vi "CallEngine.vi"(8 "error in (no error)":errorcluster, 10 "RT_Game.lvlib:Engine.lvclass":refnum<class "Engine.lvclass">, 11 "SnakeGame in":refnum<class "SnakeGame.lvclass">) -> (0 "error out":errorcluster, 2 "RT_Game.lvlib:Engine.lvclass 2":refnum<class "Engine.lvclass">, 3 "SnakeGame out":refnum<class "SnakeGame.lvclass">)   [LabVIEW 2019, in "RT_Game.lvlib" / "SnakeGame.lvclass"]
uses:
  SnakeGame.lvclass
  Engine/Engine.lvclass
  Engine/Engine.lvclass/Engine.ctl
  Engine/Write delta_t.vi
  Game/Game.lvclass
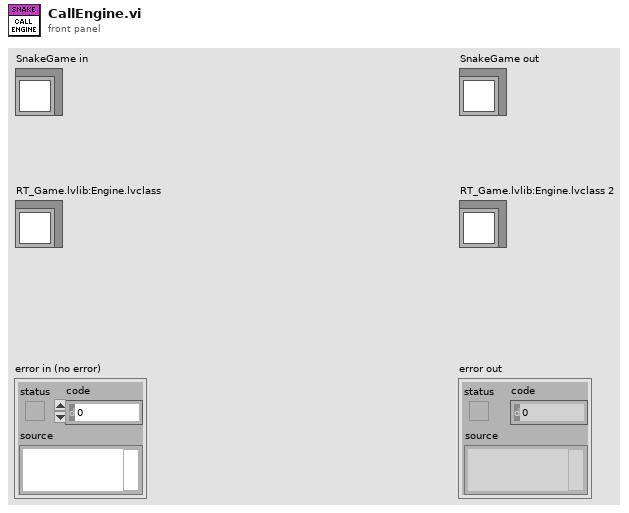
[diagram p1: front panel]
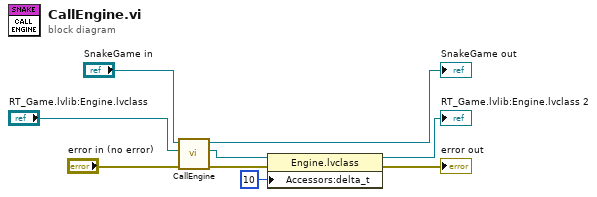
[diagram p0: block diagram]
diagram:
  n1 = call-parent "CallEngine.vi"("error in (no error)"="error in (no error)", "RT_Game.lvlib:Engine.lvclass"="RT_Game.lvlib:Engine.lvclass", "Game in"="SnakeGame in") -> ("error out"=w9:errorcluster, "RT_Game.lvlib:Engine.lvclass 2"=w3:refnum<class "Engine.lvclass">, "Game out"=→"SnakeGame out":refnum<class "SnakeGame.lvclass">)  [unwired: 6 in]
  n2 = property class="Engine.lvclass"(reference=w3, error in=w9, "Accessors:delta_t"=u16 10 ("delta_t")) -> (reference out=→"RT_Game.lvlib:Engine.lvclass 2":refnum<class "Engine.lvclass">, error out=→"error out":errorcluster)
